vi "HovaCAL Pump Concentration.vi"(11 "Water-Cluster out (Eingang)":cluster{"water conc SP":dbl, "water conc":dbl}) -> (3 "Water-Cluster out (Ausgang)":cluster{"water conc SP":dbl, "water conc":dbl})   [LabVIEW 2020, in "EPA 1065.lvlib" / "HovaCAL Interference verificaton.lvlib"]
uses:
  HovaCAL Interference verificaton.lvlib
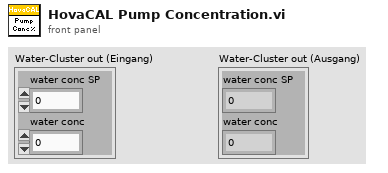
[diagram p1: front panel]
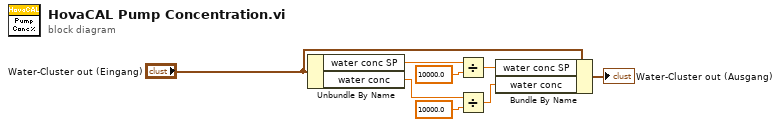
[diagram p0: block diagram]
diagram:
  n1 = Unbundle By Name("Water-Cluster out (Eingang)") -> ("water conc SP"=w2:dbl, "water conc"=w7:dbl)
  n2 = Divide(x=w2, y=10000.0) -> (x/y=w1:dbl)
  n3 = Divide(x=w7, y=10000.0) -> (x/y=w5:dbl)
  n4 = Bundle By Name(cluster="Water-Cluster out (Eingang)", "water conc SP"=w1, "water conc"=w5) -> (→"Water-Cluster out (Ausgang)":cluster{"water conc SP":dbl, "water conc":dbl})
